vi "add_CMDStatus.vi"(6 "Status":T1 {"MPC Info"."c"."3" format="%#_12g"; "MPC Info"."c"."2" format="%#_12g"; "MPC Info"."c"."1" format="%#_12g"}, 7 "msg in":string) -> (3 "msg out":string)   [LabVIEW 2018]
doc: "Flattens a pose 2D into a message"
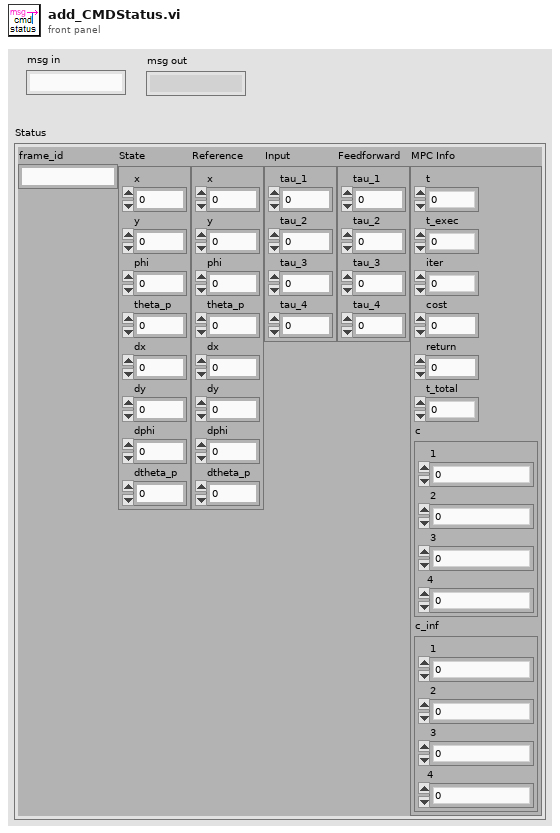
[diagram p1: front panel]
types:
  T1 = cluster{"frame_id":string, "State":cluster{"x":dbl, "y":dbl, "phi":dbl, "theta_p":dbl, "dx":dbl, "dy":dbl, "dphi":dbl, "dtheta_p":dbl}, "Reference":cluster{"x":dbl, "y":dbl, "phi":dbl, "theta_p":dbl, "dx":dbl, "dy":dbl, "dphi":dbl, "dtheta_p":dbl}, "Input":cluster{"tau_1":dbl, "tau_2":dbl, "tau_3":dbl, "tau_4":dbl}, "Feedforward":cluster{"tau_1":dbl, "tau_2":dbl, "tau_3":dbl, "tau_4":dbl}, "MPC Info":cluster{"t":dbl, "t_exec":dbl, "iter":i32, "cost":dbl, "return":i32, "t_total":dbl, "c":cluster{"1":dbl, "2":dbl, "3":dbl, "4":dbl}, "c_inf":cluster{"1":dbl, "2":dbl, "3":dbl, "4":dbl}}}
  T2 = cluster{"x":dbl, "y":dbl, "phi":dbl, "theta_p":dbl, "dx":dbl, "dy":dbl, "dphi":dbl, "dtheta_p":dbl}
  T3 = cluster{"tau_1":dbl, "tau_2":dbl, "tau_3":dbl, "tau_4":dbl}
  T4 = cluster{"t":dbl, "t_exec":dbl, "iter":i32, "cost":dbl, "return":i32, "t_total":dbl, "c":cluster{"1":dbl, "2":dbl, "3":dbl, "4":dbl}, "c_inf":cluster{"1":dbl, "2":dbl, "3":dbl, "4":dbl}}
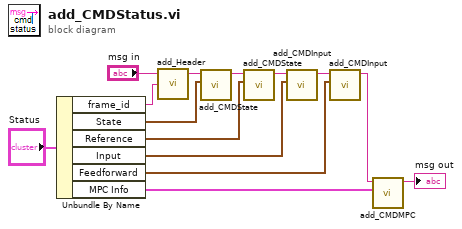
[diagram p0: block diagram]
diagram:
  n1 = Unbundle By Name("Status") -> ("frame_id"=w11:string, "State"=w10:T2, "Reference"=w7:T2, "Input"=w9:T3, "Feedforward"=w4:T3, "MPC Info"=w3:T4)
  n2 = call <userlib>:"add_Header.vi"("frame_id"=w11, "msg in"="msg in") -> ("msg out"=w14:string)  [unwired: 3 in]
  n3 = call <userlib>:"add_CMDState.vi"("State"=w10, "msg in"=w14) -> ("msg out"=w8:string)  [unwired: 5 in]
  n4 = call <userlib>:"add_CMDState.vi"("State"=w7, "msg in"=w8) -> ("msg out"=w6:string)  [unwired: 5 in]
  n5 = call <userlib>:"add_CMDInput.vi"("Input"=w9, "msg in"=w6) -> ("msg out"=w5:string)  [unwired: 5 in]
  n6 = call <userlib>:"add_CMDInput.vi"("Input"=w4, "msg in"=w5) -> ("msg out"=w2:string)  [unwired: 5 in]
  n7 = call "add_CMDMPC.vi"("MPC Info"=w3, "msg in"=w2) -> ("msg out"=→"msg out":string)  [unwired: 5 in]
